vi "Get Hub Location.vi"() -> (1 "Hub Y":dbl=4.03, 2 "Hub X":dbl)   [LabVIEW 2025]
uses:
  <vilib>/Rock Robotics/WPI/DriverStation/WPI_DriverStationAllianceInfo.ctl
panel:
  out "Alliance":T1
  in  "Hub X RED (m)":dbl=11.93800001016
  in  "Hub X BLUE (m)":dbl=4.5974
  in  "Hub Y (m)":dbl=4.03
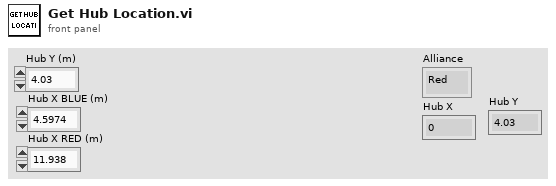
[diagram p1: front panel]
types:
  T1 = typedef "WPI_DriverStationAllianceInfo.ctl" = enum16{"Red", "Blue", "Invalid"}
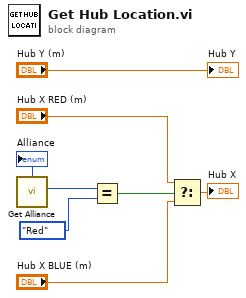
[diagram p0: block diagram]
diagram:
  n1 = call "Get Alliance.vi"() -> ("Alliance"=w6:T1)  [unwired: 11 in]
  "Alliance" <- w6
  n2 = Equal?(x=w6, y=WPI_DriverStationAllianceInfo."Red") -> (x = y?=w3:bool)
  n3 = Select(t="Hub X RED (m)", s=w3, f="Hub X BLUE (m)") -> (s? t:f=→"Hub X":dbl)
  "Hub Y" <- "Hub Y (m)"
